vi "Poista Debuger VI.vi"(8 "error in (no error)":errorcluster, 11 "Actor in":refnum<class "Actor.lvclass">) -> (0 "error out":errorcluster, 3 "Actor out":refnum<class "Actor.lvclass">)   [LabVIEW 2015]
uses:
  <vilib>/ActorFramework/Actor/Actor.lvclass
  CO2 Actor.lvclass
panel:
  out "error out 2":errorcluster
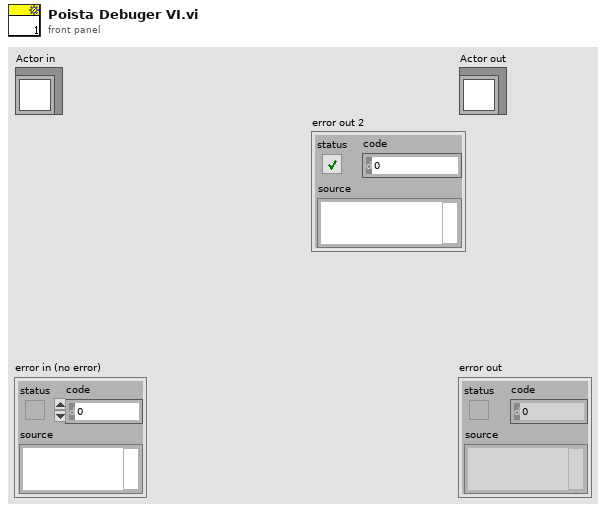
[diagram p1: front panel]
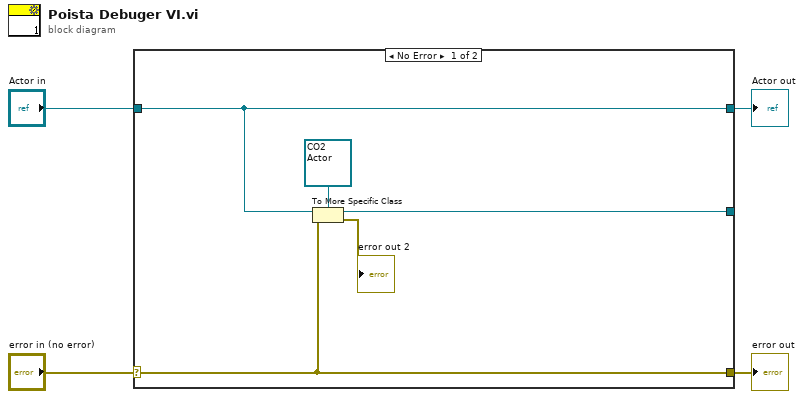
[diagram p0: block diagram]
diagram:
  n1 = case shown="No Error" "error in (no error)" {
    selector: "error in (no error)" -> [w6 w11]
    tunnel: [w6 w11] -> w3
    tunnel: [w9 w10] -> w1
    tunnel: "Actor in" -> [w9 w10]
    tunnel: [w7 _] -> _
    frame No Error {
      n2 = To More Specific Class(target class=refnum<class "CO2 Actor.lvclass"> refnum ("CO2 Actor.lvclass"), reference=w9, error in=w6) -> (specific class reference=w7:refnum<class "CO2 Actor.lvclass">, error out=→"error out 2":errorcluster)
    }
    frame Error {
    }
  }
  "error out" <- w3
  "Actor out" <- w1
